vi "_magnitude_to_dB.vi"(0 "Lin Mag in":cluster{dbl[], dbl[]}) -> (1 "Cluster":cluster{dbl[], dbl[]}, 2 "Freq":dbl[](array[numeric]), 3 "dB":dbl[](array[numeric]), 4 "ArrayVersion":dbl[][](array[numeric]))   [LabVIEW 2013]
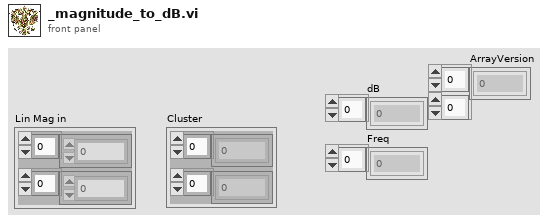
[diagram p1: front panel]
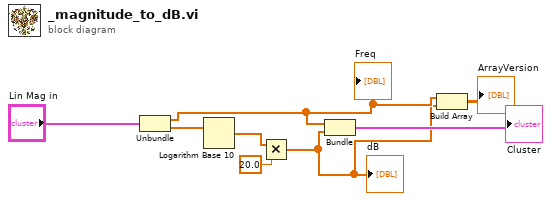
[diagram p0: block diagram]
diagram:
  n1 = Unbundle("Lin Mag in") -> (w3:dbl[], w6:dbl[])
  "Freq" <- w3
  n2 = Logarithm Base 10(1:w6) -> (0:w8:dbl[])
  n3 = Multiply(x=w8, y=20.0 ("x")) -> (x*y=w2:dbl[])
  "dB" <- w2
  n4 = Bundle(w3, w2) -> (→"Cluster":cluster{dbl[], dbl[]})  [unwired: 1 in]
  n5 = Build Array(w3, w2) -> (→"ArrayVersion":dbl[][])
